vi "FTW-Message-Request-Body.vi"(8 "error in":errorcluster, 11 "FTW Incoming Request":refnum<class "FTW-Message-IncomingRequest.lvclass">) -> (0 "error out":errorcluster, 1 "Request Body":string, 3 "FTW Incoming Request out":refnum<class "FTW-Message-IncomingRequest.lvclass">)   [LabVIEW 2013, in "FTW-Message-IncomingRequest.lvclass"]
uses:
  FTW-Message-IncomingRequest.lvclass
panel:
  # "Inputs"
  # "Outputs"
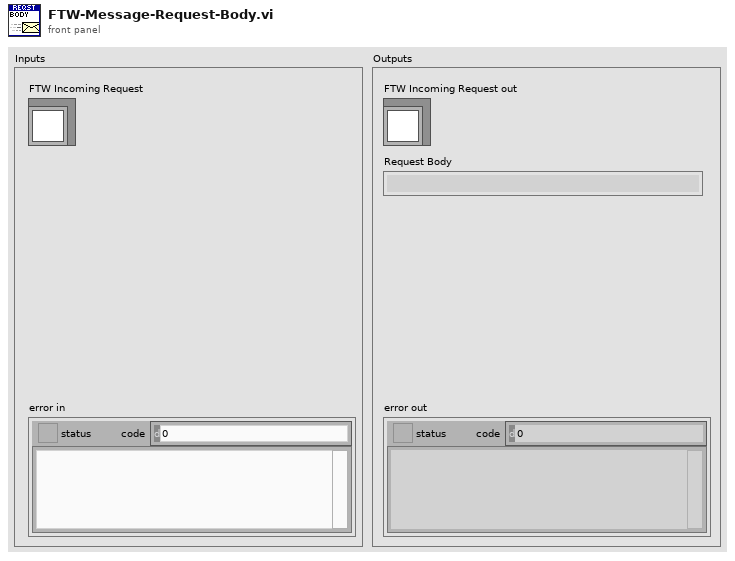
[diagram p1: front panel]
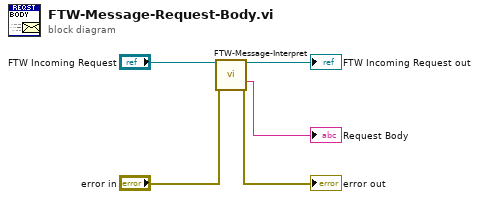
[diagram p0: block diagram]
diagram:
  n1 = call-dynamic "FTW-Message-Interpret.vi"("FTW Message"="FTW Incoming Request", "error in"="error in") -> ("FTW Message out"=→"FTW Incoming Request out":refnum<class "FTW-Message-IncomingRequest.lvclass">, "Message Body"=→"Request Body":string, "error out"=→"error out":errorcluster)  [unwired: 9 in, 2 out]
